vi "Process 2.vi"(8 "error in (no error)":errorcluster, 9 "Data B queue":refnum<queue>, 10 "Data A queue":refnum<queue>, 11 "Stop notifier":refnum<notifier>) -> (0 "error out":errorcluster)   [LabVIEW 2012]
uses:
  Data type A.ctl
  Data type B.ctl
  <vilib>/Platform/TimedLoop/XDataNode/timing_clust.ctl
  <vilib>/Platform/TimedLoop/XDataNode/nitl_modes.ctl
  <vilib>/Platform/TimedLoop/XDataNode/wakeup.ctl
  <vilib>/Platform/TimedLoop/XDataNode/XDataNode.xnode
  <vilib>/Platform/TimedLoop/XDataNode/XDNodeRunTimeDep.lvlib
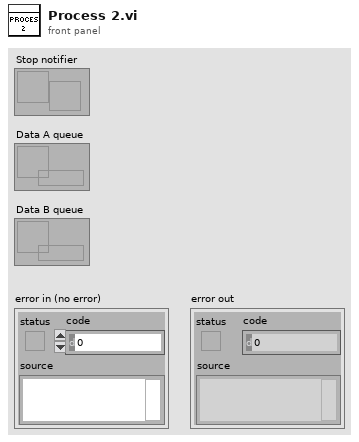
[diagram p1: front panel]
types:
  T1 = typedef "XDNodeRunTimeDep.lvlib/timing_clust.ctl" = cluster{"Expected End [f-1]":u64, "Actual End [f-1]":u64, "Finished Late? [f-1]":bool, "Expected End [i-1]":u64, "Actual End [i-1]":u64, "Finished Late? [i-1]":bool, "Expected Start [i]":u64, "Actual Start [i]":u64, "Expected Start [f]":u64, "Actual Start [f]":u64, "Source Name":string, "Structure Name":string, "Period":i64, "Deadline":i64, "Offset":i64, "Start":i64, "Priority":i32, "Timeout":i32, "Mode":T2, "Wakeup Reason":T3, "Error":errorcluster, "Source Type":string, "Secondary Source Type":string, "Global End Time":u64, "Global Start Time":u64, "Frame Duration":u64, "Iteration Duration":u64, "Assigned CPU":i32, "I/O Scan Engine Mode":u32}
  T2 = typedef "XDNodeRunTimeDep.lvlib/nitl_modes.ctl" = enum32{"No Change", "Process missed periods, maintain original phase", "Discard missed periods, maintain original phase", "Process missed periods, ignore original phase", "Discard missed periods, ignore original phase"}
  T3 = typedef "XDNodeRunTimeDep.lvlib/wakeup.ctl" = enum32{"Normal", "Aborted", "Asynchronous wakeup", "Timing source error", "Timed loop error", "Timeout"}
  T4 = typedef "Data type B.ctl" = cluster{"Numeric":dbl, "Boolean":bool}
  T5 = typedef "Data type A.ctl" = dbl
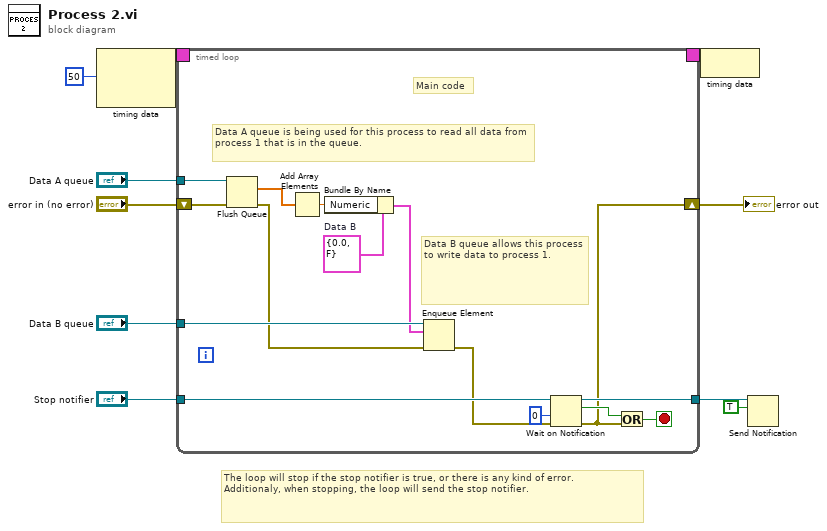
[diagram p0: block diagram]
diagram:
  # "The loop will stop if the stop notifier is true, or there is any kind of error.\nAdditionaly, when stopping, the loop will send the stop notifier."
  n1 = node-c288(i64 50 ("Period")) -> (w10:T1)  [unwired: 1 in]
  n2 = timed-loop {
    timing: w10 -> [_]
    timing-out: [_] -> w9
    tunnel: "Data A queue" -> [w24]
    tunnel: "Data B queue" -> [w25]
    shift-right: [w11] -> w1
    shift-left: "error in (no error)" -> [w19]
    tunnel: "Stop notifier" -> [w16]
    tunnel: [w13] -> w3
    stop <- w14 stop-if-true
    w22 = T4 {"Numeric"=0.0, "Boolean"=FALSE}  # Data B
    # "Data B queue allows this process to write data to process 1."
    # "Data A queue is being used for this process to read all data from process 1 that is in the queue."
    # "Main code"
    n3 = Flush Queue(queue=w24, error in (no error)=w19) -> (remaining elements=w23:T5[], error out=w18:errorcluster)  [unwired: 1 out]
    n4 = Add Array Elements(numeric array=w23) -> (sum=w21:T5)
    n5 = Bundle By Name(cluster=w22, "Numeric"=w21) -> (w20:T4)
    n6 = Enqueue Element(queue=w25, element=w20, error in (no error)=w18) -> (error out=w12:errorcluster)  [unwired: 1 in, 2 out]
    n7 = Wait on Notification(notifier=w16, timeout in ms (-1)=0, error in (no error)=w12) -> (notifier out=w13:refnum<notifier>, notification=w15:bool, error out=w11:errorcluster)  [unwired: 1 in, 1 out]
    n8 = Or(x=w15, y=w11) -> (x .or. y?=w14:bool)
  }
  "error out" <- w1
  n9 = node-c288(w9) -> ()
  n10 = Send Notification(notification=TRUE, notifier=w3) -> ()  [unwired: 1 in, 2 out]
